vi "Get FlexLogger Configuration.vi"(8 "error in (no error)":errorcluster) -> (0 "error out":errorcluster, 3 "Local FlexLogger Configuration":refnum<class "NI Skyline Configuration AMQP.lvclass">)   [LabVIEW 2020, in "FlexLoggerTagHelpers.lvlib"]
uses:
  FlexLoggerTagHelpers.lvlib
  <vilib>/Skyline/Configuration/Configuration_class/NI Skyline Configuration.lvclass
  <vilib>/Skyline/Configuration/Configuration AMQP_class/Open Configuration AMQP.vi
  <vilib>/Skyline/Configuration/Configuration AMQP_class/NI Skyline Configuration AMQP.lvclass
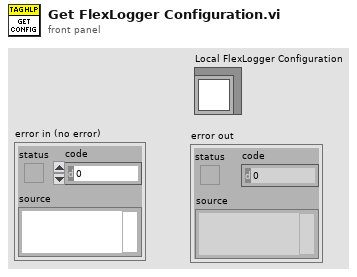
[diagram p1: front panel]
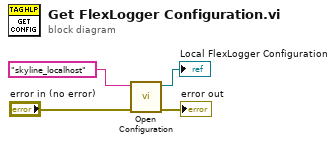
[diagram p0: block diagram]
diagram:
  n1 = call-poly <vilib>:"Open Configuration.vi"("error in (no error)"="error in (no error)", "configuration id"="skyline_localhost") -> ("error out"=→"error out":errorcluster, "configuration"=→"Local FlexLogger Configuration":refnum<class "NI Skyline Configuration AMQP.lvclass">)  [unwired: 8 in]
